vi "Initialize Monitoring Channels.vi"(8 "error in (no error)":errorcluster, 11 "VeriStand Data Sharing Framework in":refnum<class "VeriStand DSF.lvclass">) -> (0 "error out":errorcluster, 3 "VeriStand Data Sharing Framework out":refnum<class "VeriStand DSF.lvclass">)   [LabVIEW 2020, in "DSF Engine.lvlib" / "VeriStand DSF.lvclass"]
uses:
  VeriStand DSF.lvclass
  VeriStand DSF.lvclass/VeriStand DSF.ctl
  <vilib>/NI VeriStand/Custom Device API/Data Access Type.ctl
  DSF Core.lvlibp/Typedefs/DSF Data Type.ctl
  DSF Core.lvlibp/Classes/Buffer/Buffer.lvclass
  <vilib>/NI VeriStand/Custom Device API/Custom Device API.lvlib
  DSF Shared.lvlib
  DSF Core.lvlibp/Classes/Framework/Framework.lvclass
  Source/DSF Core.lvlibp
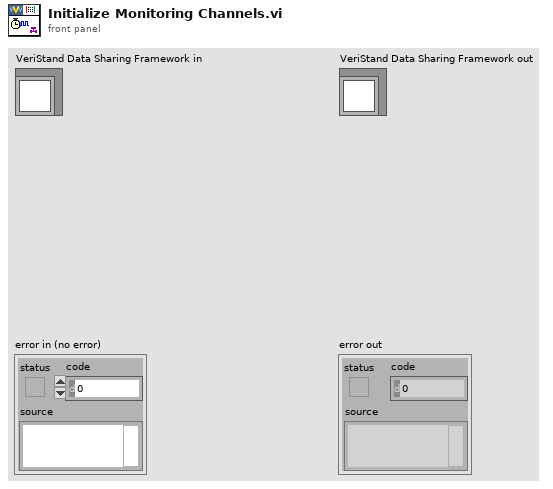
[diagram p1: front panel]
types:
  T1 = typedef "Custom Device API.lvlib/Custom Device Item Ref.ctl" = u64
  T2 = typedef "Custom Device API.lvlib/Data Access Type.ctl" = enum16{"Read", "Write"}
  T3 = typedef "DSF Core.lvlibp/DSF Data Type.ctl" = enum8{"Bool", "SGL", "DBL", "I8", "I16", "I32", "I64", "U8", "U16", "U32", "U64"}
  T4 = typedef "Custom Device API.lvlib/Data Reference.ctl" = i32
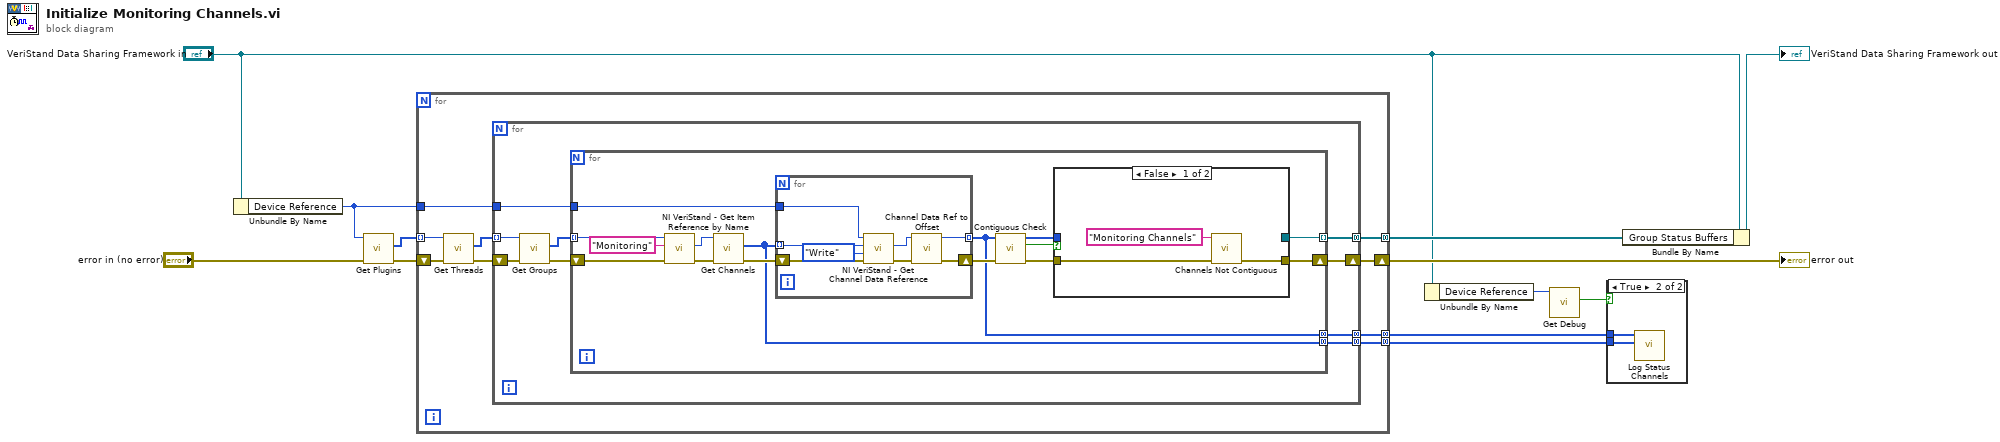
[diagram p0: block diagram]
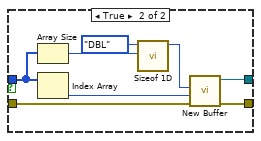
[diagram p2: hidden frame]
diagram:
  n1 = Unbundle By Name("VeriStand Data Sharing Framework in") -> ("Device Reference"=w7:T1)
  n2 = call "Get Plugins.vi"("error in (no error)"="error in (no error)", "Item Ref in"=w7) -> ("error out"=w12:errorcluster, "Plugin refs"=w11:T1[])  [unwired: 7 in, 1 out]
  n3 = for {
    tunnel: w11 -> [w18] mode=indexing
    tunnel: w7 -> [w20]
    shift-right: [w21] -> w2
    shift-left: w12 -> [w19]
    tunnel: [w15] -> w9 mode=concatenating
    tunnel: [w14] -> w5 mode=concatenating
    tunnel: [w13] -> w4 mode=concatenating
    n4 = call "Get Threads.vi"("error in (no error)"=w19, "Item Ref in"=w18) -> ("error out"=w17:errorcluster, "Plugin refs"=w16:T1[])  [unwired: 7 in, 1 out]
    n5 = for {
      tunnel: w16 -> [w27] mode=indexing
      tunnel: w20 -> [w30]
      shift-right: [w29] -> w21
      shift-left: w17 -> [w28]
      tunnel: [w24] -> w15 mode=concatenating
      tunnel: [w23] -> w14 mode=concatenating
      tunnel: [w22] -> w13 mode=concatenating
      n6 = call "Get Groups.vi"("error in (no error)"=w28, "Plugin Ref in"=w27) -> ("error out"=w26:errorcluster, "Group refs"=w25:T1[])  [unwired: 7 in, 1 out]
      n7 = for {
        tunnel: w25 -> [w32] mode=indexing
        tunnel: w30 -> [w45]
        shift-right: [w40] -> w29
        shift-left: w26 -> [w34]
        tunnel: [w39] -> w24 mode=indexing
        tunnel: [w36] -> w23 mode=concatenating
        tunnel: [w38] -> w22 mode=concatenating
        n8 = call <vilib>:"NI VeriStand - Get Item Reference by Name.vi"("error in (no error)"=w34, "Item Name"="Monitoring", "Parent Ref in"=w32) -> ("error out"=w33:errorcluster, "Item Ref"=w31:T1)  [unwired: 5 in, 2 out]
        n9 = call "Get Channels.vi"("error in (no error)"=w33, "Item Ref in"=w31) -> ("error out"=w37:errorcluster, "Channels refs"=w36:T1[])  [unwired: 7 in, 1 out]
        n10 = for {
          shift-right: [w52] -> w44
          shift-left: w37 -> [w51]
          tunnel: [w49] -> w38 mode=indexing
          tunnel: w45 -> [w47]
          tunnel: w36 -> [w46] mode=indexing
          n11 = call <vilib>:"NI VeriStand - Get Channel Data Reference.vi"("error in (no error)"=w51, "Access"=Data_Access_Type."Write", "Channel Ref in"=w46, "Device Ref in"=w47) -> ("error out"=w53:errorcluster, "Channel Data Reference"=w50:T4)  [unwired: 5 in, 1 out]
          n12 = call "Channel Data Ref to Offset.vi"("error in (no error)"=w53, "Channel Data Reference"=w50) -> ("error out"=w52:errorcluster, "channel offset"=w49:u64)  [unwired: 8 in]
        }
        n13 = call "Contiguous Check.vi"("error in (no error)"=w44, "channel offsets in"=w38) -> ("error out"=w43:errorcluster, "contiguous?"=w42:bool, "channel offsets out"=w41:u64[])  [unwired: 7 in]
        n14 = case shown="False" w42 {
          tunnel: w43 -> [w56 w64]
          tunnel: w41 -> [_ w60]
          tunnel: [w55 w57] -> w40
          tunnel: [_ w58] -> w39
          frame False {
            n15 = call "Channels Not Contiguous.vi"("error in (no error)"=w56, "name"="Monitoring Channels") -> ("error out"=w55:errorcluster)  [unwired: 9 in]
          }
          frame True {
            n16 = Array Size(array=w60) -> (size(s)=w63:i32)
            n17 = Index Array(array=w60) -> (element=w61:u64)  [unwired: 1 in]
            n18 = call "Sizeof 1D.vi"("count"=w63, "data type"=DSF_Data_Type."DBL") -> ("size in bytes"=w59:u64)  [unwired: 9 in]
            n19 = call "New Buffer.vi"("error in (no error)"=w64, "buffer offset (0)"=w61, "buffer size"=w59) -> ("error out"=w57:errorcluster, "Buffer out"=w58:refnum<class "Buffer.lvclass">)  [unwired: 7 in]
          }
        }
      }
    }
  }
  "error out" <- w2
  n20 = Unbundle By Name("VeriStand Data Sharing Framework in") -> ("Device Reference"=w6:T1)
  n21 = call "Get Debug.vi"("Item Ref in"=w6) -> ("debug"=w3:bool)  [unwired: 8 in, 2 out]
  n22 = case shown="True" w3 {
    tunnel: w5 -> [_ w66]
    tunnel: w4 -> [_ w65]
    frame False {
    }
    frame True {
      n23 = call "Log Status Channels.vi"("status channels refs"=w66, "status channel offsets"=w65) -> ()  [unwired: 10 in]
    }
  }
  n24 = Bundle By Name(cluster="VeriStand Data Sharing Framework in", "Group Status Buffers"=w9) -> (→"VeriStand Data Sharing Framework out":refnum<class "VeriStand DSF.lvclass">)
